vi "stop daemon.vi"(8 "error in (no error)":errorcluster) -> (0 "error out":errorcluster)   [LabVIEW 2016, in "数据传输系统-06.lvlib" / "update.lvlib"]
uses:
  update.lvlib
panel:
  out "standard error":string caption="标准错误"
  out "standard output":string caption="标准输出"
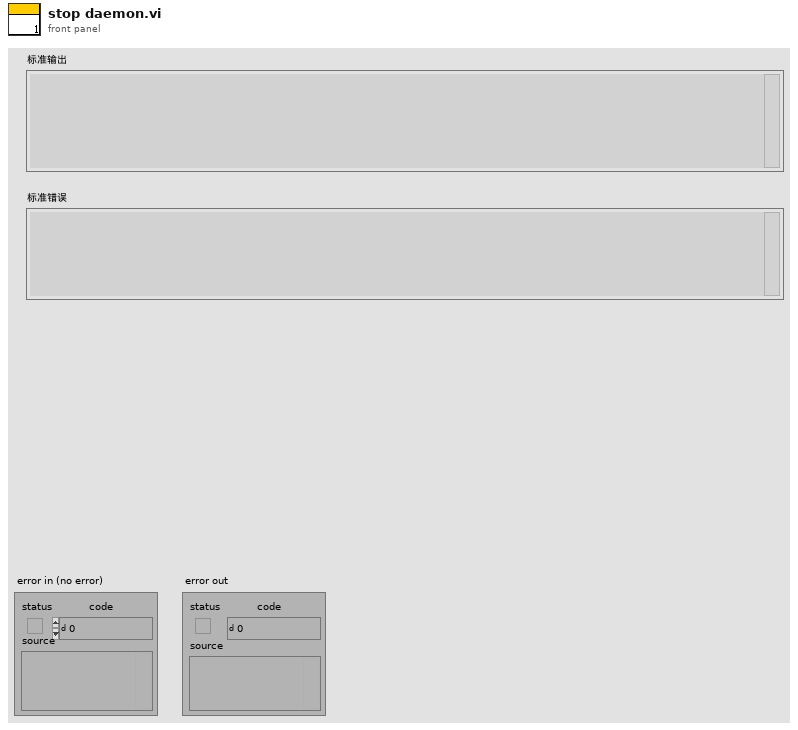
[diagram p1: front panel]
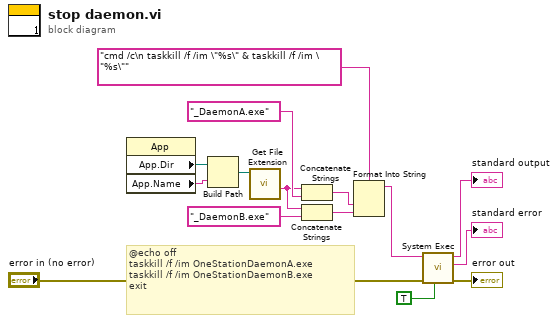
[diagram p0: block diagram]
diagram:
  # "@echo off\ntaskkill /f /im OneStationDaemonA.exe\ntaskkill /f /im OneStationDaemonB.exe\nexit"
  n1 = property class="App"() -> ("App.Dir"=w3:path, "App.Name"=w2:string)  [unwired: 2 in, 2 out]
  n2 = Build Path(base path=w3, name or relative path=w2) -> (appended path=w1:path)
  n3 = call <vilib>:"Get File Extension.vi"("file"=w1) -> ("filename without extension"=w12:string)  [unwired: 6 in, 4 out]
  n4 = Concatenate Strings(w12, "_DaemonA.exe" ("名称或相对路径")) -> (w11:string)
  n5 = Concatenate Strings(w12, "_DaemonB.exe" ("名称或相对路径")) -> (w10:string)
  n6 = Format Into String(format string="cmd /c\n taskkill /f /im \"%s\" & taskkill /f /im \"%s\"" ("格式字符串"), w11, w10) -> (resulting string=w9:string)  [unwired: 2 in, 1 out]
  n7 = call <vilib>:"System Exec.vi"("run minimized? (F)"=TRUE, "error in (no error)"="error in (no error)", "command line"=w9) -> ("error out"=→"error out":errorcluster, "standard error"=→"standard error":string, "standard output"=→"standard output":string)  [unwired: 5 in, 1 out]
